vi "Test Log Warning Message.vi"(8 "error in (no error)":errorcluster, 11 "Test Case In":refnum<class "Logger Test.lvclass">) -> (0 "error out":errorcluster, 3 "Test Case Out":refnum<class "Logger Test.lvclass">)   [LabVIEW 2020, in "Logger Test.lvclass"]
uses:
  Logger Test.lvclass
  Mock Log Handler/Mock Log Handler.lvclass
  Framework/Process/Process.lvclass
  Mock Process/Mock Process.lvclass
  <vilib>/Asteme/LUnit/Test Case.lvclass
  C:/Program Files (x86)/National Instruments/LabVIEW 2020/vi.lib/Asteme/LUnit/Test Case.lvclass
  C:/Users/anton/Documents/GitHub/Triarc-Framework/source/Framework Test/Logger Test/Logger Test.lvclass
  C:/Users/anton/Documents/GitHub/Triarc-Framework/source/Framework/Process/Process.lvclass
  C:/Users/anton/Documents/GitHub/Triarc-Framework/source/Framework/Base/Base.lvclass
  C:/Users/anton/Documents/GitHub/Triarc-Framework/source/Framework/Error Handler Interface/Error Handler Interface.lvclass
  C:/Users/anton/Documents/GitHub/Triarc-Framework/source/Framework/Logging/Logging.lvclass
  C:/Users/anton/Documents/GitHub/Triarc-Framework/source/Framework Test/Mock Process/Mock Process.lvclass
  C:/Users/anton/Documents/GitHub/Triarc-Framework/source/Framework/Helper Loop/Helper Loop.lvclass
  Framework/Logging/Logging.lvclass
  C:/Users/anton/Documents/GitHub/Triarc-Framework/source/Framework Test/Mock Log Handler/Mock Log Handler.lvclass
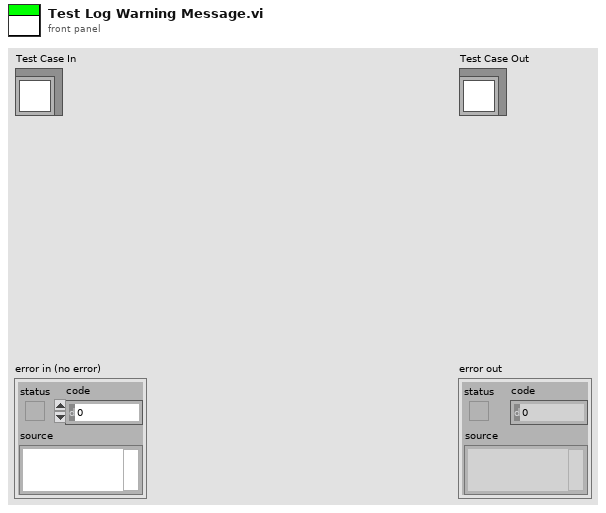
[diagram p1: front panel]
types:
  T1 = typedef "Mock Log Handler.lvclass/Log Entry.ctl" = cluster{"Level":string, "Source":string, "Message":string}
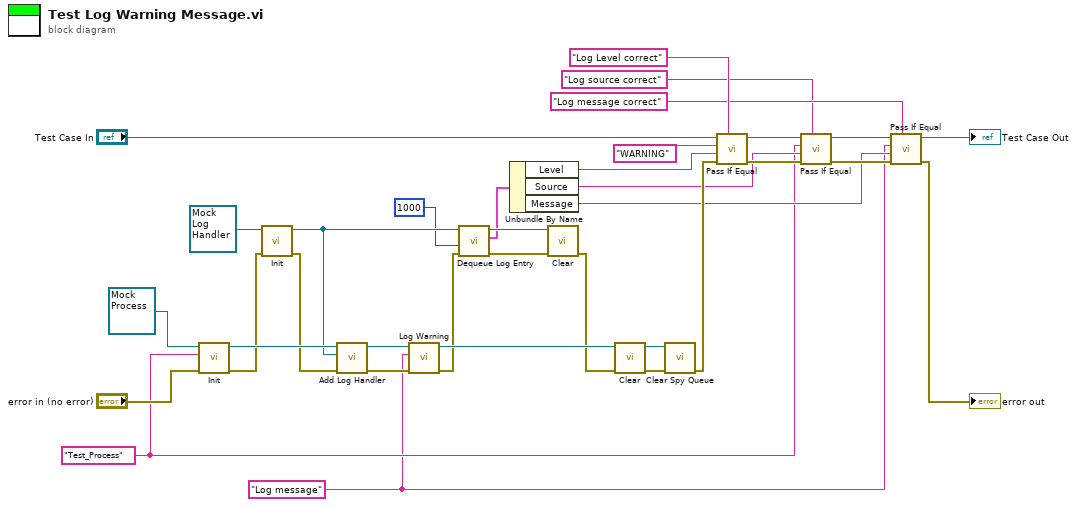
[diagram p0: block diagram]
diagram:
  w1 = "Log message" ("Message")
  w2 = "Test_Process" ("Name")
  n1 = call-dynamic "Init.vi"("error in (no error)"="error in (no error)", "Name"=w2, "Mock Process In"=refnum<class "Mock Process.lvclass"> refnum) -> ("error out"=w25:errorcluster, "Mock Process Out"=w32:refnum<class "Mock Process.lvclass">)  [unwired: 7 in]
  n2 = call-dynamic "Init.vi"("error in (no error)"=w25, "Mock Log Handler In"=refnum<class "Mock Log Handler.lvclass"> refnum ("Mock Log Handler.lvclass")) -> ("error out"=w24:errorcluster, "Mock Log Handler Out"=w21:refnum<class "Mock Log Handler.lvclass">)  [unwired: 8 in]
  n3 = call "Add Log Handler.vi"("error in (no error)"=w24, "Log Handler"=w21, "Process In"=w32) -> ("error out"=w31:errorcluster, "Process Out"=w19:refnum<class "Mock Process.lvclass">)  [unwired: 7 in]
  n4 = call "Log Warning.vi"("error in (no error)"=w31, "Message"=w1, "Logging In"=w19) -> ("error out"=w17:errorcluster, "Logging Out"=w18:refnum<class "Mock Process.lvclass">)  [unwired: 7 in]
  n5 = call "Dequeue Log Entry.vi"("error in (no error)"=w17, "timeout in ms (-1)"=1000, "Mock Log Handler in"=w21) -> ("error out"=w22:errorcluster, "Entry"=w15:T1, "Mock Log Handler out"=w23:refnum<class "Mock Log Handler.lvclass">)  [unwired: 5 in, 1 out]
  n6 = Unbundle By Name(w15) -> ("Level"=w14:string, "Source"=w4:string, "Message"=w3:string)
  n7 = call-dynamic "Clear.vi"("error in (no error)"=w22, "Mock Log Handler In"=w23) -> ("error out"=w16:errorcluster)  [unwired: 8 in, 1 out]
  n8 = call-dynamic "Clear.vi"("error in (no error)"=w16, "Mock Process In"=w18) -> ("error out"=w29:errorcluster, "Mock Process Out"=w30:refnum<class "Mock Process.lvclass">)  [unwired: 8 in]
  n9 = call-dynamic "Clear Spy Queue.vi"("error in (no error)"=w29, "Mock Process In"=w30) -> ("error out"=w8:errorcluster)  [unwired: 8 in, 1 out]
  n10 = call <vilib>:"Pass If Equal.vi"("Description"="Log Level correct", "error in (no error)"=w8, "Actual"=w14, "Expected"="WARNING", "Test Case In"="Test Case In") -> ("error out"=w10:errorcluster, "Test Case Out"=w34:refnum<class "Logger Test.lvclass">)  [unwired: 5 in]
  n11 = call <vilib>:"Pass If Equal.vi"("Description"="Log source correct", "error in (no error)"=w10, "Actual"=w4, "Expected"=w2, "Test Case In"=w34) -> ("error out"=w9:errorcluster, "Test Case Out"=w12:refnum<class "Logger Test.lvclass">)  [unwired: 5 in]
  n12 = call <vilib>:"Pass If Equal.vi"("Description"="Log message correct", "error in (no error)"=w9, "Actual"=w3, "Expected"=w1, "Test Case In"=w12) -> ("error out"=→"error out":errorcluster, "Test Case Out"=→"Test Case Out":refnum<class "Logger Test.lvclass">)  [unwired: 5 in]
